vi "Simple Execute.vi"(1 "Report":refnum<class "Report.lvclass">, 8 "error in (no error)":errorcluster, 9 "Parameters":refnum<class "PropertyObject.lvclass">, 10 "Entry Point / Sequence":string, 11 "SequenceFile in":refnum<class "SequenceFile.lvclass">) -> (0 "error out":errorcluster, 2 "Status":string, 3 "SequenceFile out":refnum<class "SequenceFile.lvclass">)   [LabVIEW 2020, in "TSnax.lvlib" / "SequenceFile.lvclass"]
uses:
  SequenceFile.lvclass
  SequenceFile.lvclass/SequenceFile.ctl
  PropertyObject/PropertyObject.lvclass
  Report/Report.lvclass
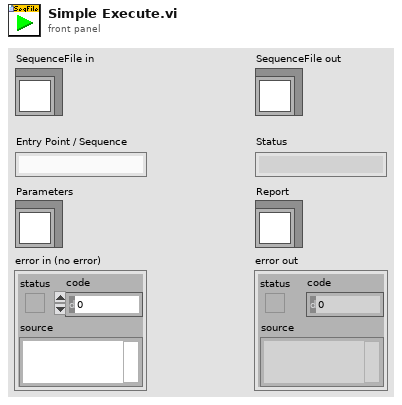
[diagram p1: front panel]
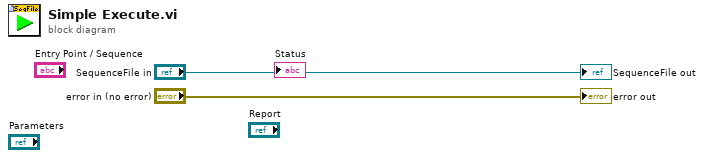
[diagram p0: block diagram]
diagram:
  "error out" <- "error in (no error)"
  "SequenceFile out" <- "SequenceFile in"
